vi "Test GenNet-Client API.vi"() -> ()   [LabVIEW 2020]
doc: "GenNet-Client API Tester.\n\n____\nHAMPEL SOFTWARE ENGINEERING v3.8.0 (2023-12-18 14:41)"
uses:
  <vilib>/Utility/error.llb/DialogType.ctl
  DQMH-GenNet Message Queue.lvclass
  hse-dqmh/Controls/System Message Argument--cluster.ctl
  hse-dqmh/Controls/System Message Source.ctl
  DQMH-GenNet Message Queue.lvclass/DQMH-GenNet Message Queue.ctl
  GenNet-Client.lvlib
  hse-dqmh/hse-dqmh.lvlib
panel:
  out "last error":errorcluster
  in  "Multicast Address":string
  in  "Port":u16
  in  "Listen for Network Broadcasts":bool
  in  "Connect":bool
  in  "Timeout":i32
  in  "Port No.":u16
  in  "IP Address":string
  in  "message":string
  in  "Message Data":variant
  in  "Send":bool
  in  "Run as Singleton?":bool
  in  "Show Block Diagram":bool
  in  "Refresh Modules":bool
  out "Active Modules":string[](array[string])
  in  "Stop Module":bool
  in  "Select Module":i32(ring)=-1 caption="Select Module\nTo send Request to" items=["All"=-1]
  in  "Run New Module":bool
  in  "Hide Module Panel":bool
  in  "Show Module Panel":bool
  out "Status":string
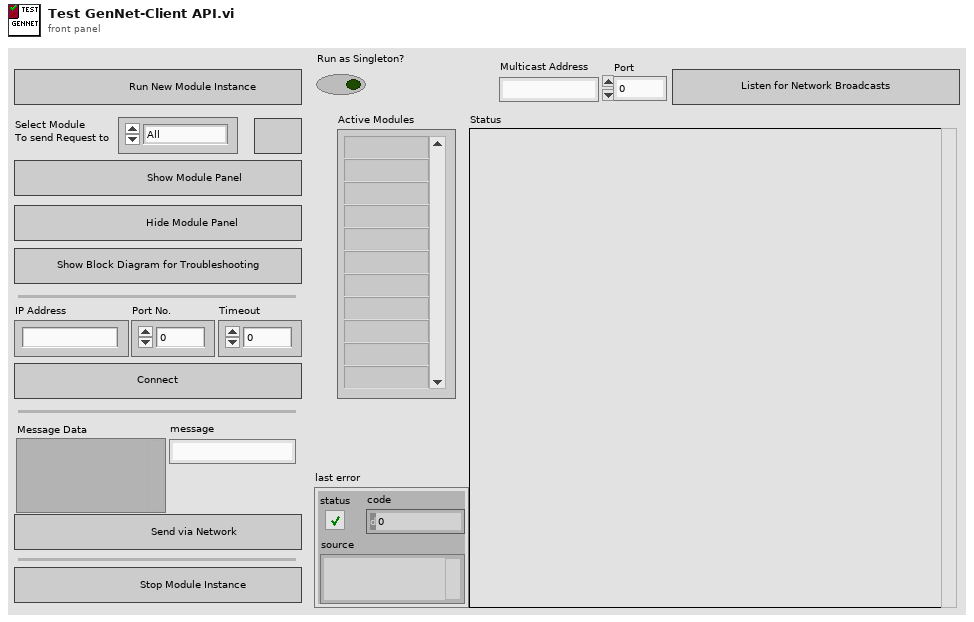
[diagram p1: front panel]
types:
  T1 = typedef "GenNet-Client.lvlib/Broadcast Events--cluster.ctl" = cluster{"Module Did Init":refnum<user-event>, "Status Updated":refnum<user-event>, "Error Reported":refnum<user-event>, "Module Did Stop":refnum<user-event>, "Update Module Execution Status":refnum<user-event>}
  T2 = typedef "DialogType.ctl" = u16
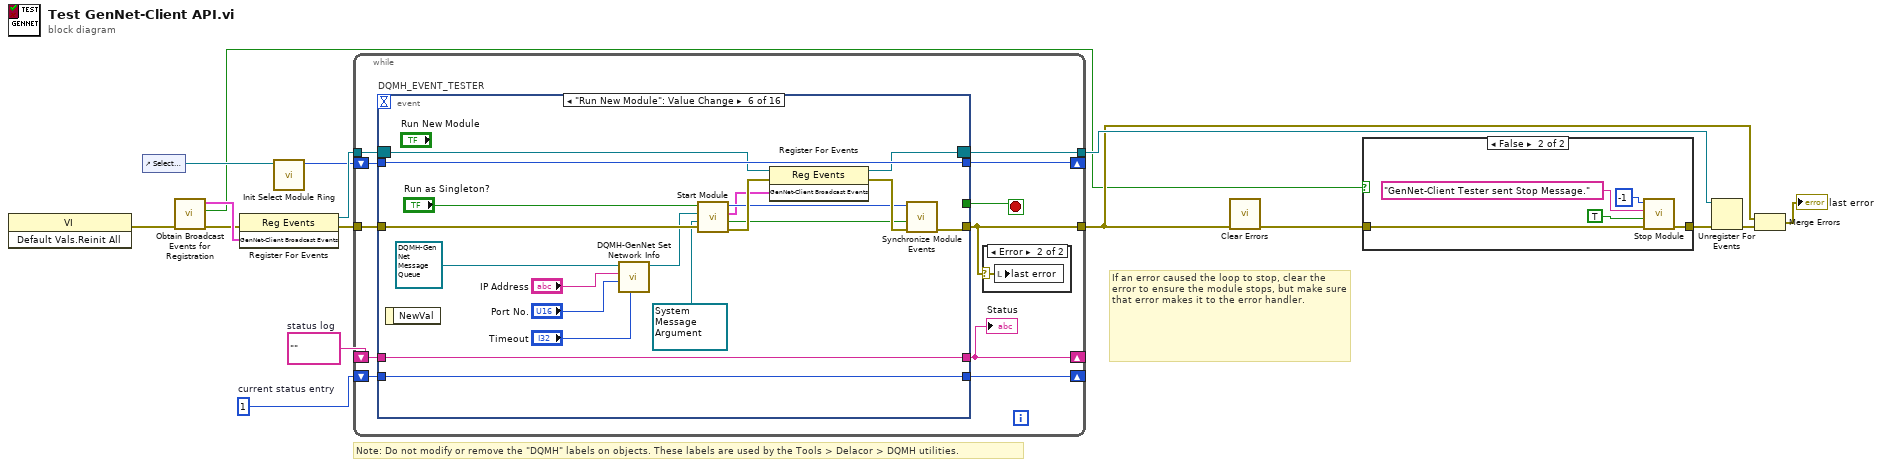
[diagram p0: block diagram]
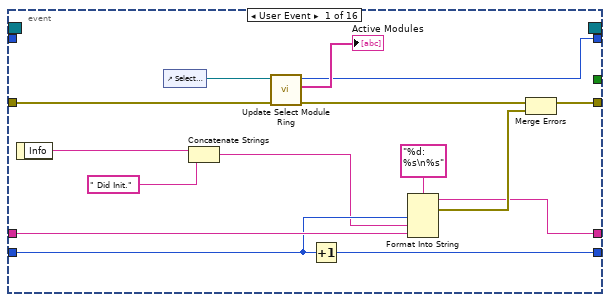
[diagram p4: hidden frame]
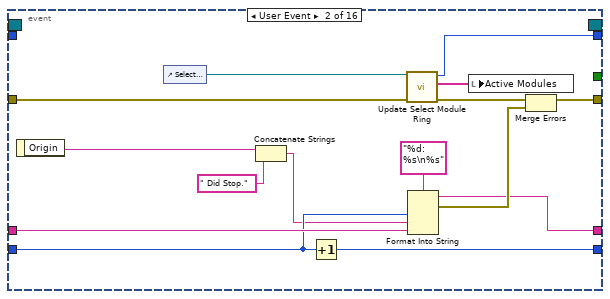
[diagram p5: hidden frame]
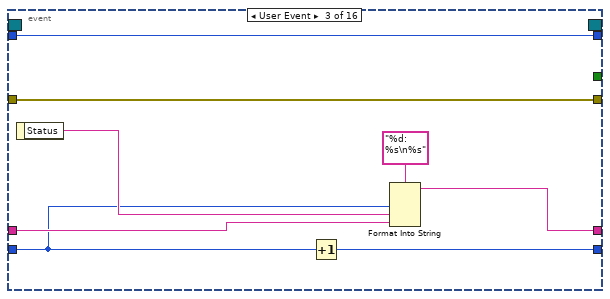
[diagram p6: hidden frame]
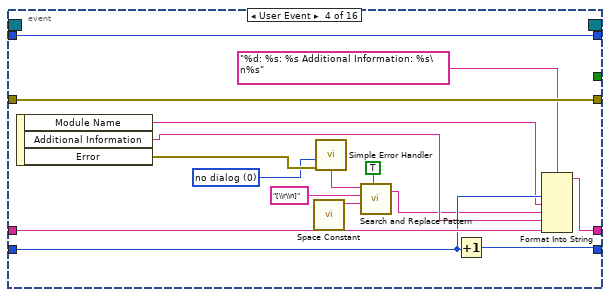
[diagram p7: hidden frame]
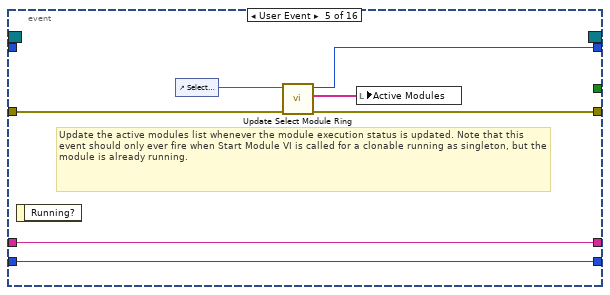
[diagram p8: hidden frame]
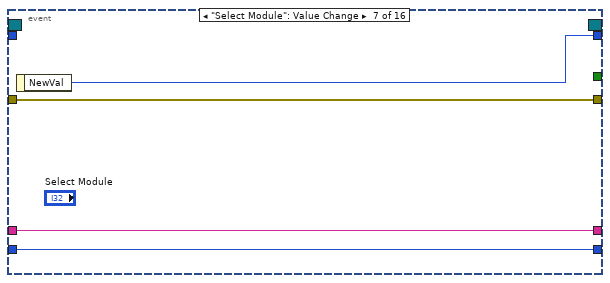
[diagram p9: hidden frame]
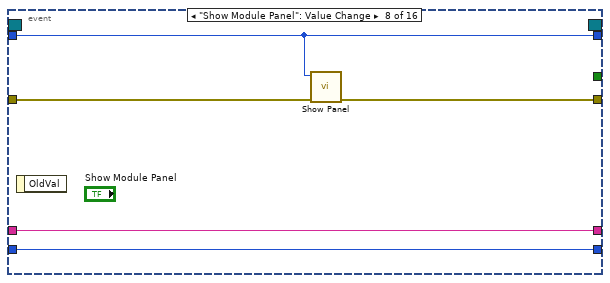
[diagram p10: hidden frame]
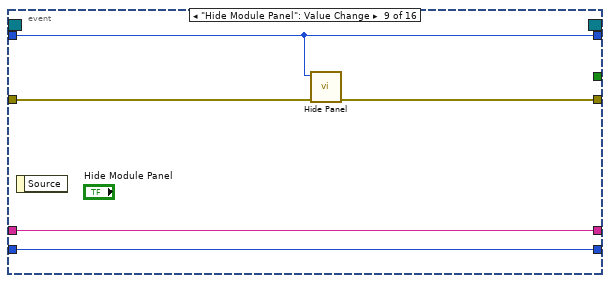
[diagram p11: hidden frame]
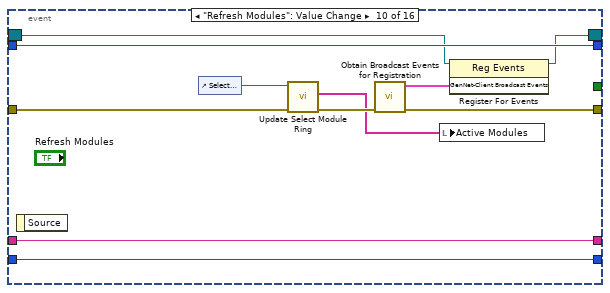
[diagram p12: hidden frame]
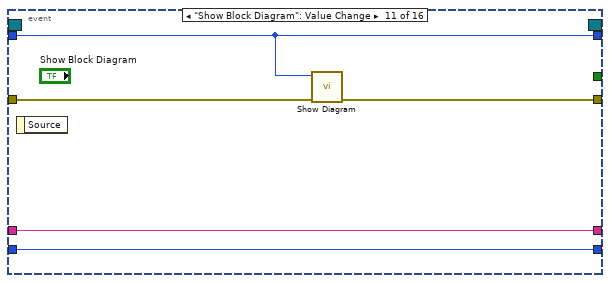
[diagram p13: hidden frame]
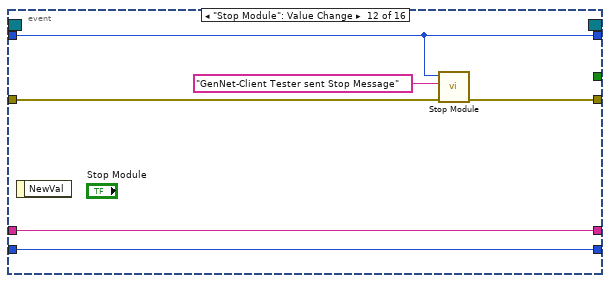
[diagram p14: hidden frame]
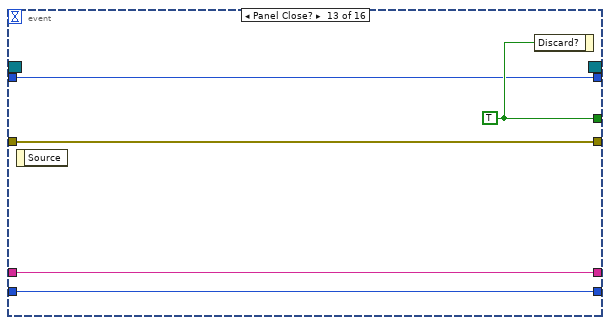
[diagram p15: hidden frame]
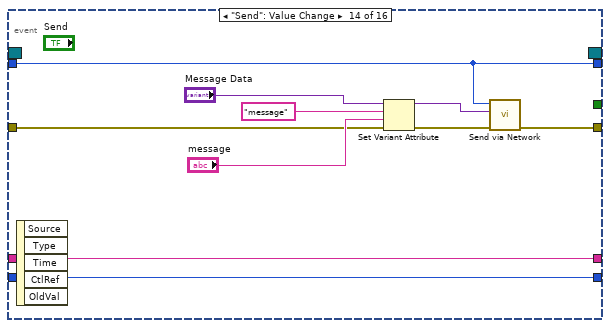
[diagram p16: hidden frame]
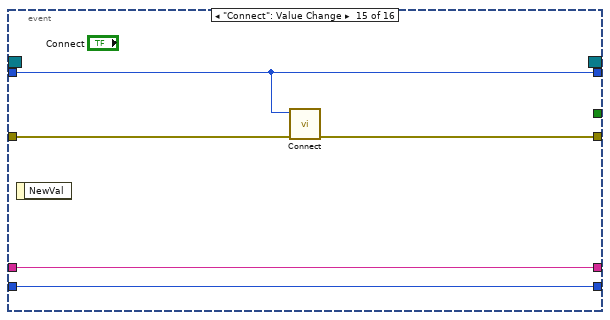
[diagram p17: hidden frame]
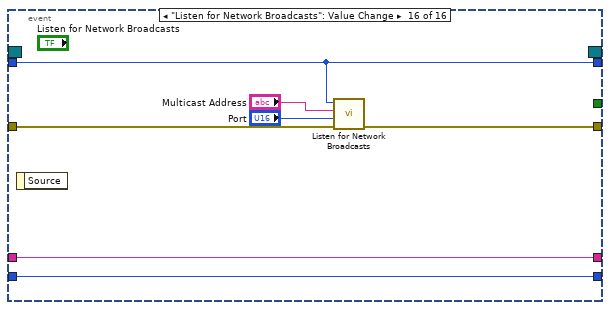
[diagram p18: hidden frame]
diagram:
  w12 = 1  # current status entry
  w13 = ""  # status log
  # "If an error caused the loop to stop, clear the error to ensure the module stops, but make sure that error makes it to the error handler."
  # "Note: Do not modify or remove the \"DQMH\" labels on objects. These labels are used by the Tools > Delacor > DQMH utilities."
  n1 = invoke class="VI" method="Default Vals.Reinit All"() -> (error out=w4:errorcluster)  [unwired: 3 in, 2 out]
  n2 = control-ref of="Select Module"() -> (w10:refnum<vi>)
  n3 = call "Obtain Broadcast Events for Registration.vi"("error in (no error)"=w4) -> ("error out"=w3:errorcluster, "Already running?"=w2:bool, "GenNet-Client Broadcast Events"=w9:T1)  [unwired: 8 in]
  n4 = register-events(error in=w3, w9) -> (reference out=w16:refnum<event-registration>, error out=w8:errorcluster)  [unwired: 1 in]
  n5 = call "Init Select Module Ring.vi"("Select Module Ring Ref"=w10) -> ("Value for All Modules"=w11:i32)  [unwired: 8 in, 2 out]
  n6 = while {
    tunnel: w16 -> [w27]
    tunnel: [w18] -> w5
    tunnel: w8 -> [w26]
    shift-right: [w22] -> _
    shift-left: w13 -> [w24]
    shift-right: [w23] -> _
    shift-left: w12 -> [w25]
    shift-right: [w20] -> _
    shift-left: w11 -> [w21]
    tunnel: [w19] -> w7
    stop <- w17 stop-if-true
    n7 = event "DQMH_EVENT_TESTER" shown="[5] \"Run New Module\": Value Change" {
      selector: w27 -> [_ _ _ _ _ w102 _ _ _ w128 _ _ _ _ _ _]
      dyn-events: [_ _ _ _ _ w101 _ _ _ w127 _ _ _ _ _ _] -> w19
      timeout: _ -> [_ _ _ _ _ _ _ _ _ _ _ _ _ _ _ _]
      tunnel: [_ _ _ _ _ _ _ _ _ _ _ _ w149 _ _ _] -> w17
      tunnel: [w32 w50 w66 w81 w85 w100 w112 w116 w121 w124 w135 w140 w148 w157 w161 w168] -> w18
      tunnel: w26 -> [w34 w52 w66 w81 w86 w103 w112 w117 w122 w129 w138 w141 w148 w151 w164 w171]
      tunnel: w25 -> [w40 w55 w59 w78 w88 w105 w110 w114 w119 w132 w136 w143 w146 w158 w162 w169]
      tunnel: w24 -> [w41 w56 w62 w80 w89 w106 w111 w115 w120 w133 w137 w144 w147 w159 w163 w170]
      tunnel: [w38 w53 w63 w79 w89 w106 w111 w115 w120 w133 w137 w144 w147 w159 w163 w170] -> w22
      tunnel: [w39 w54 w65 w77 w88 w105 w110 w114 w119 w132 w136 w143 w146 w158 w162 w169] -> w23
      tunnel: w21 -> [_ _ w60 w82 _ w104 _ w113 w118 w131 w134 w142 w145 w156 w160 w167]
      tunnel: [w29 w47 w60 w82 w84 w104 w109 w113 w118 w131 w134 w142 w145 w156 w160 w167] -> w20
      event User Event {
        n8 = event-data() -> ("Info"=w37:string)  [unwired: 1 in]
        n9 = control-ref of="Select Module"() -> (w31:refnum<vi>)
        n10 = Concatenate Strings(w37, " Did Init.") -> (w36:string)
        n11 = call "Update Select Module Ring.vi"("error in (no error)"=w34, "Select Module Ring Ref"=w31) -> ("error out"=w33:errorcluster, "Active Modules (Array)"=→"Active Modules":string[], "New Module Ring Value"=w29:i32)  [unwired: 7 in]
        n12 = Increment(x=w40) -> (x+1=w39:i32)
        n13 = Format Into String(format string="%d: %s\n%s", w40, w36, w41) -> (resulting string=w38:string, error out=w43:errorcluster)  [unwired: 2 in]
        n14 = Merge Errors(w33, w43) -> (w32:errorcluster)
      }
      event User Event {
        n15 = event-data() -> ("Origin"=w45:string)  [unwired: 1 in]
        n16 = control-ref of="Select Module"() -> (w49:refnum<vi>)
        n17 = Concatenate Strings(w45, " Did Stop.") -> (w44:string)
        n18 = Increment(x=w55) -> (x+1=w54:i32)
        n19 = call "Update Select Module Ring.vi"("error in (no error)"=w52, "Select Module Ring Ref"=w49) -> ("error out"=w51:errorcluster, "Active Modules (Array)"=w48:string[], "New Module Ring Value"=w47:i32)  [unwired: 7 in]
        n20 = Format Into String(format string="%d: %s\n%s", w55, w44, w56) -> (resulting string=w53:string, error out=w58:errorcluster)  [unwired: 2 in]
        n21 = local write "Active Modules"(w48) -> ()
        n22 = Merge Errors(w51, w58) -> (w50:errorcluster)
      }
      event User Event {
        n23 = event-data() -> ("Status"=w61:string)  [unwired: 1 in]
        n24 = Increment(x=w59) -> (x+1=w65:i32)
        n25 = Format Into String(format string="%d: %s\n%s", w59, w61, w62) -> (resulting string=w63:string)  [unwired: 2 in, 1 out]
      }
      event User Event {
        w73 = T2 0 items=["no dialog", "OK message", "continue or stop message", "OK message + warnings", "continue/stop + warnings"] ("type of dialog (OK msg:1)")
        n26 = event-data() -> ("Module Name"=w74:string, "Additional Information"=w75:string, "Error"=w76:errorcluster)  [unwired: 1 in]
        n27 = call <vilib>:"Space Constant.vi"() -> ("String"=w69:string)
        n28 = call <vilib>:"Simple Error Handler.vi"("type of dialog (OK msg:1)"=w73, "error in (no error)"=w76) -> ("message"=w72:string)  [unwired: 3 in, 4 out]
        n29 = call <vilib>:"Search and Replace Pattern.vi"("string"=w72, "regular expression (\"\")"="[\\r\\n]" ("regular expression (\"\")"), "replace string (\"\")"=w69, "replace all? (F)"=TRUE ("replace all CR/LF with spaces")) -> ("result string"=w71:string)  [unwired: 1 in, 1 out]
        n30 = Increment(x=w78) -> (x+1=w77:i32)
        n31 = Format Into String(format string="%d: %s: %s Additional Information: %s\n%s", w78, w74, w71, w75, w80) -> (resulting string=w79:string)  [unwired: 2 in, 1 out]
      }
      event User Event {
        # "Update the active modules list whenever the module execution status is updated. Note that this event should only ever fire when Start Module VI is called for a clonable running as singleton, but the module is already running."
        n32 = event-data() -> ()  [unwired: 1 in, 1 out]
        n33 = control-ref of="Select Module"() -> (w87:refnum<vi>)
        n34 = call "Update Select Module Ring.vi"("error in (no error)"=w86, "Select Module Ring Ref"=w87) -> ("error out"=w85:errorcluster, "Active Modules (Array)"=w83:string[], "New Module Ring Value"=w84:i32)  [unwired: 7 in]
        n35 = local write "Active Modules"(w83) -> ()
      }
      event "Run New Module": Value Change {
        n36 = event-data() -> ()  [unwired: 1 in, 1 out]
        n37 = call "DQMH-GenNet Set Network Info.vi"("Timeout (default 5000ms)"="Timeout", "Port Number"="Port No.", "IP Address"="IP Address", "Message Queue in"=refnum<class "DQMH-GenNet Message Queue.lvclass"> refnum ("Caller MsgQ")) -> ("Message Queue out"=w94:refnum<class "DQMH-GenNet Message Queue.lvclass">)  [unwired: 6 in, 1 out]
        n38 = call "Start Module.vi"("error in (no error)"=w103, "Caller SystemMsg"=refnum<user-event> refnum, "Caller MsgQ"=w94, "Run as Singleton? (F)"="Run as Singleton?") -> ("error out"=w107:errorcluster, "Wait for Event Sync?"=w98:bool, "GenNet-Client Broadcast Events"=w97:T1, "Module ID"=w99:i32)  [unwired: 4 in]
        n39 = register-events(reference=w102, error in=w107, w97) -> (reference out=w101:refnum<event-registration>, error out=w108:errorcluster)
        n40 = call "Synchronize Module Events.vi"("error in (no error)"=w108, "Wait for Event Sync?"=w98, "Module ID"=w99) -> ("error out"=w100:errorcluster)  [unwired: 7 in, 1 out]
      }
      event "Select Module": Value Change {
        n41 = event-data() -> ("NewVal"=w109:i32)  [unwired: 1 in]
      }
      event "Show Module Panel": Value Change {
        n42 = event-data() -> ()  [unwired: 1 in, 1 out]
        n43 = call "Show Panel.vi"("error in (no error)"=w117, "Module ID"=w113) -> ("error out"=w116:errorcluster)  [unwired: 9 in]
      }
      event "Hide Module Panel": Value Change {
        n44 = event-data() -> ()  [unwired: 1 in, 1 out]
        n45 = call "Hide Panel.vi"("error in (no error)"=w122, "Module ID"=w118) -> ("error out"=w121:errorcluster)  [unwired: 9 in]
      }
      event "Refresh Modules": Value Change {
        n46 = event-data() -> ()  [unwired: 1 in, 1 out]
        n47 = control-ref of="Select Module"() -> (w130:refnum<vi>)
        n48 = call "Update Select Module Ring.vi"("error in (no error)"=w129, "Select Module Ring Ref"=w130) -> ("error out"=w125:errorcluster, "Active Modules (Array)"=w123:string[])  [unwired: 7 in, 1 out]
        n49 = call "Obtain Broadcast Events for Registration.vi"("error in (no error)"=w125) -> ("error out"=w124:errorcluster, "GenNet-Client Broadcast Events"=w126:T1)  [unwired: 8 in, 1 out]
        n50 = local write "Active Modules"(w123) -> ()
        n51 = register-events(reference=w128, w126) -> (reference out=w127:refnum<event-registration>)  [unwired: 1 in, 1 out]
      }
      event "Show Block Diagram": Value Change {
        n52 = event-data() -> ()  [unwired: 1 in, 1 out]
        n53 = call "Show Diagram.vi"("error in (no error)"=w138, "Module ID"=w134) -> ("error out"=w135:errorcluster)  [unwired: 9 in]
      }
      event "Stop Module": Value Change {
        n54 = event-data() -> ()  [unwired: 1 in, 1 out]
        n55 = call "Stop Module.vi"("error in (no error)"=w141, "Origin"="GenNet-Client Tester sent Stop Message", "Module ID"=w142) -> ("error out"=w140:errorcluster)  [unwired: 8 in]
      }
      event Panel Close? {
        w149 = TRUE ("Discard?")
        n56 = event-data() -> ()  [unwired: 1 in, 1 out]
        n57 = event-data("Discard?"=w149) -> ()  [unwired: 1 in, 1 out]
      }
      event "Send": Value Change {
        n58 = event-data() -> ()  [unwired: 1 in, 5 out]
        n59 = Set Variant Attribute(Variant="Message Data", name="message", value="message", error in=w151) -> (Variant out=w154:variant, error out=w150:errorcluster)  [unwired: 1 out]
        n60 = call "Send via Network.vi"("error in (no error)"=w150, "Message Data"=w154, "Module ID"=w156) -> ("error out"=w157:errorcluster)  [unwired: 8 in]
      }
      event "Connect": Value Change {
        n61 = event-data() -> ()  [unwired: 1 in, 1 out]
        n62 = call "Connect.vi"("error in (no error)"=w164, "Module ID"=w160) -> ("error out"=w161:errorcluster)  [unwired: 8 in, 1 out]
      }
      event "Listen for Network Broadcasts": Value Change {
        n63 = event-data() -> ()  [unwired: 1 in, 1 out]
        n64 = call "Listen for Network Broadcasts.vi"("error in (no error)"=w171, "Port"="Port", "Multicast Address"="Multicast Address", "Module ID"=w167) -> ("error out"=w168:errorcluster)  [unwired: 7 in]
      }
    }
    "Status" <- w22
    n65 = case "DQMH_TESTER_ERROR_LOCAL" shown="Error" w18 {
      selector: w18 -> [_ w28]
      frame No Error {
      }
      frame Error {
        n66 = local write "last error"(w28) -> ()
      }
    }
  }
  n67 = call <vilib>:"Clear Errors.vi"("error in (no error)"=w5) -> ("error out"=w6:errorcluster)  [unwired: 5 in, 1 out]
  n68 = case shown="False" w2 {
    tunnel: [w172 w177] -> w14
    tunnel: w6 -> [w172 w174]
    frame True {
    }
    frame False {
      n69 = call "Stop Module.vi"("error in (no error)"=w174, "Wait for Module to stop? (F)"=TRUE ("Wait for Module to stop?"), "Origin"="GenNet-Client Tester sent Stop Message.", "Module ID"=-1) -> ("error out"=w177:errorcluster)  [unwired: 7 in]
    }
  }
  n70 = Unregister For Events(event registration refnum=w7, error in=w14) -> (error out=w15:errorcluster)
  n71 = Merge Errors(w5, w15) -> (→"last error":errorcluster)
